vi "LVClass_Pupil Load Data.vi"(0 "Pupil in":refnum<class "Pupil.lvclass">, 5 "file path txt":path, 11 "error in (no error)":errorcluster) -> (4 "Pupil out":refnum<class "Pupil.lvclass">, 15 "error out":errorcluster)   [LabVIEW 2020, in "Pupil.lvclass"]
doc: "Set Pupil buffer.\n\n--------------------------------------------------------------------------------\n\n<B>PupilIn </B> : Pupil object.\n<B>PupilOut </B> : Pupil object.\n<B>data </B> : Pupil buffer to set.\n<B>ErrorIn </B> : Error\n<B>ErrorOut </B> : Error\n\n--------------------------------------------------------------------------------"
uses:
  Pupil.lvclass
  Pupil.lvclass/Pupil.ctl
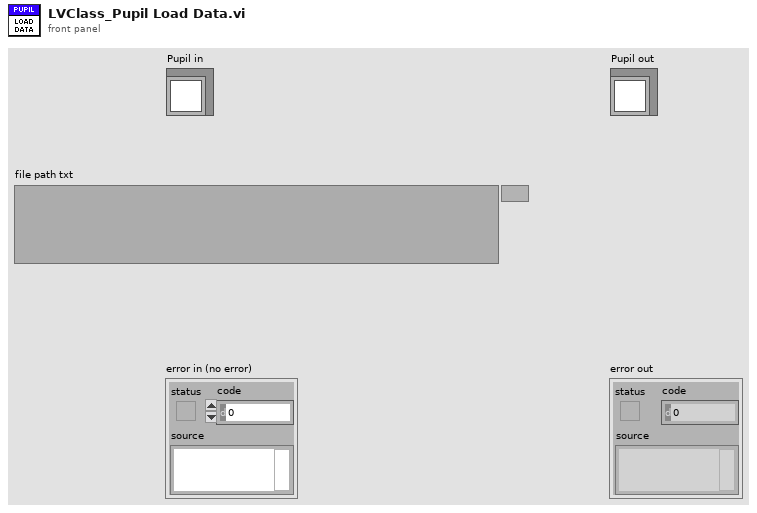
[diagram p1: front panel]
types:
  T1 = typedef "ClassID.ctl" = i64
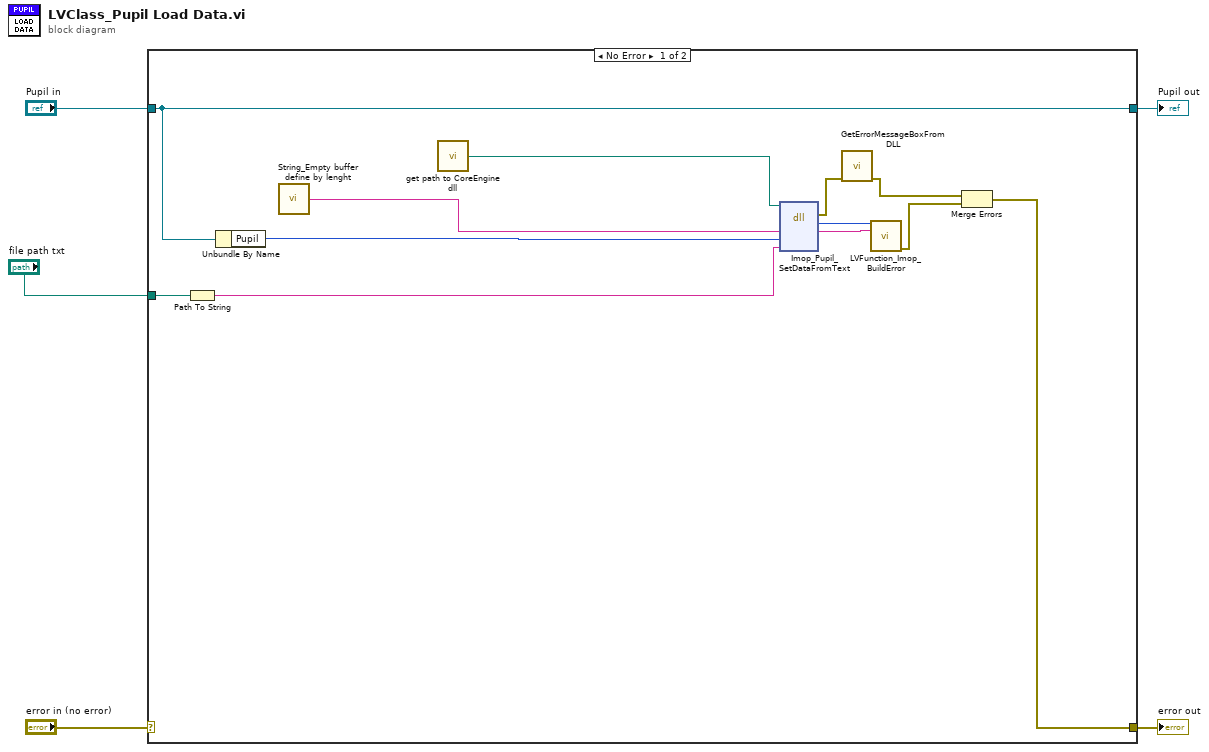
[diagram p0: block diagram]
diagram:
  n1 = case shown="No Error" "error in (no error)" {
    selector: "error in (no error)" -> [_ w19]
    tunnel: [w8 w19] -> w5
    tunnel: [w12 w18] -> w4
    tunnel: "Pupil in" -> [w12 w18]
    tunnel: "file path txt" -> [w7 _]
    frame No Error {
      n2 = Path To String(path=w7) -> (string=w6:string)
      n3 = Unbundle By Name(w12) -> ("Pupil"=w11:T1)
      n4 = call "String_Empty buffer define by lenght.vi"() -> ("Empty buffer"=w17:string)  [unwired: 1 in]
      n5 = call "get path to CoreEngine dll.vi"() -> ("path to wavekit library"=w14:path)  [unwired: 14 in, 1 out]
      n6 = dll-call lib="D:/2_trunk/Soft_haso/ImOpCoreEngine4_LV2011/DLLs/ImopEngine4_vc100.dll" fn="Imop_Pupil_SetDataFromText"(path in=w14, "message"=w17, "objet"=w11, "Data"=w6) -> (error out=w13:errorcluster, "return type"=w15:i32, "message"=w16:string)  [unwired: 4 in, 1 out]
      n7 = call "GetErrorMessageBoxFromDLL.vi"("error IN"=w13) -> ("error OUT"=w10:errorcluster)  [unwired: 10 in]
      n8 = call "LVFunction_Imop_BuildError.vi"("code"=w15, "String to Prepend to source (\"\")"=w16) -> ("error out"=w9:errorcluster)  [unwired: 13 in]
      n9 = Merge Errors(w10, w9) -> (w8:errorcluster)
    }
    frame Error {
    }
  }
  "error out" <- w5
  "Pupil out" <- w4
